vi "UNITEST MAIN v2.0.vi"() -> ()   [LabVIEW 2025] (continued)
      n79 = Bundle By Name(cluster=w163, "Loading.Enter the Loading Rate (N/min)"=w161, "Loading.Message"=w160, "Loading.Warning 2"=w159, "Loading.SSP 0.75"=w158, "Loading.SSP 0.5"=w157, "Loading.SSP 0.3"=w156, "Loading.Warning"=w155, "Loading.gui GIF"=w154, "Loading.Communication is established"=w153, "Loading.AppLoad 4"=w152, "Loading.Multipoint"=w151, "Loading.Indentation"=w150, "Loading.Reference Sample"=w149, "Loading.Load Cell Communication Slide"=w148, "Loading.com 3"=w147, "Loading.com"=w146, "Loading.DecaForce COM Status"=w145, "Loading.Update"=w144, "Loading.Clear 3"=w143, "Loading.seq"=w142, "Loading.Stribeck table"=w141, "Loading.Stribeck Table  For loading"=w140, "Loading.Loading Mode"=w139, "Loading.Enter the Final Load (N)"=w138, "Loading.Enter the CoF Trip"=w137, "Loading.Enter the Friction Force Trip"=w136, "Loading.Enter the Normal load Trip"=w135, "Loading.Enter the Load  (N)"=w134, "Loading.KiloForce"=w133, "Loading.DecaForce"=w132, "Loading.MicroForce"=w131, "Loading.LHBack"=w130, "Loading.LHNext"=w129, "Loading.Load Selection"=w128) -> (w162:T22)
    }
    frame #5 {
      n80 = control-ref of="TEST SELECTION"() -> (w215:refnum<vi>)
      n81 = control-ref of="SPEED SELECTION :"() -> (w214:refnum<vi>)
      n82 = control-ref of="SPEED SELECTION : rotary"() -> (w181:refnum<vi>)
      n83 = control-ref of="Rotary Tab"() -> (w230:refnum<vi>)
      n84 = control-ref of="e.v/ssr 2"() -> (w227:refnum<vi>)
      n85 = control-ref of="Step Speed"() -> (w211:refnum<vi>)
      n86 = control-ref of="M3 Image"() -> (w206:refnum<vi>)
      n87 = control-ref of="Rotary Module Selection"() -> (w183:refnum<vi>)
      n88 = control-ref of="zNL"() -> (w232:refnum<vi>)
      n89 = control-ref of="E.Velocity 2"() -> (w228:refnum<vi>)
      n90 = control-ref of="Ramp Up 2"() -> (w216:refnum<vi>)
      n91 = control-ref of="Angular Oscillation Set"() -> (w213:refnum<vi>)
      n92 = control-ref of="Traction"() -> (w212:refnum<vi>)
      n93 = control-ref of="Surge Forward MM"() -> (w208:refnum<vi>)
      n94 = control-ref of="Surge Backward MM"() -> (w207:refnum<vi>)
      n95 = control-ref of="Sway Left MM"() -> (w204:refnum<vi>)
      n96 = control-ref of="Sway Right MM"() -> (w203:refnum<vi>)
      n97 = control-ref of="Disable Axis Jog Soft Limits"() -> (w202:refnum<vi>)
      n98 = control-ref of="Heave Down MM"() -> (w200:refnum<vi>)
      n99 = control-ref of="Heave Up MM"() -> (w199:refnum<vi>)
      n100 = control-ref of="Set WTD"() -> (w197:refnum<vi>)
      n101 = control-ref of="HomeScratch"() -> (w196:refnum<vi>)
      n102 = control-ref of="HomeRot"() -> (w195:refnum<vi>)
      n103 = control-ref of="PlaceModule"() -> (w194:refnum<vi>)
      n104 = control-ref of="LR Sway"() -> (w190:refnum<vi>)
      n105 = control-ref of="Rot Hor"() -> (w189:refnum<vi>)
      n106 = control-ref of="Scratch"() -> (w188:refnum<vi>)
      n107 = control-ref of="LR Cam"() -> (w187:refnum<vi>)
      n108 = control-ref of="MMBack"() -> (w186:refnum<vi>)
      n109 = control-ref of="MMNext"() -> (w185:refnum<vi>)
      n110 = control-ref of="Rot Ver"() -> (w184:refnum<vi>)
      n111 = control-ref of="calculate rotary"() -> (w182:refnum<vi>)
      n112 = control-ref of="Import 2"() -> (w180:refnum<vi>)
      n113 = control-ref of="Save 2"() -> (w179:refnum<vi>)
      n114 = control-ref of="SwaySpeed Set"() -> (w172:refnum<vi>)
      n115 = control-ref of="HomeScratch"() -> (w168:refnum<vi>)
      n116 = control-ref of="NL disp"() -> (w231:refnum<vi>)
      n117 = control-ref of="Enter Fixed E.Velocity 2"() -> (w226:refnum<vi>)
      n118 = control-ref of="Enter Final SRR 2"() -> (w225:refnum<vi>)
      n119 = control-ref of="Enter initial SRR 2"() -> (w224:refnum<vi>)
      n120 = control-ref of="Enter Fixed SRR 2"() -> (w223:refnum<vi>)
      n121 = control-ref of="Enter the Final E.Velocity (m/s) 2"() -> (w222:refnum<vi>)
      n122 = control-ref of="Enter initial E.Velocity (m/s) 2"() -> (w221:refnum<vi>)
      n123 = control-ref of="Final Speed (RPM) 3"() -> (w220:refnum<vi>)
      n124 = control-ref of="Initial Speed (RPM) 2"() -> (w219:refnum<vi>)
      n125 = control-ref of="Enter the Final Velocity (m/s) 3"() -> (w218:refnum<vi>)
      n126 = control-ref of="Enter initial Velocity (m/s)  3"() -> (w217:refnum<vi>)
      n127 = control-ref of="mm"() -> (w201:refnum<vi>)
      n128 = control-ref of="Wear Track Diameter (mm)"() -> (w198:refnum<vi>)
      n129 = control-ref of="Enter the Angle (Deg)"() -> (w193:refnum<vi>)
      n130 = control-ref of="Enter the Frequency (Hz)"() -> (w192:refnum<vi>)
      n131 = control-ref of="Enter the Speed(mm/sec)"() -> (w175:refnum<vi>)
      n132 = control-ref of="Enter the Speed (RPM)"() -> (w174:refnum<vi>)
      n133 = control-ref of="Enter Scratch Speed (mm/s):"() -> (w173:refnum<vi>)
      n134 = control-ref of="Scartch Offset"() -> (w171:refnum<vi>)
      n135 = control-ref of="Enter Scratch length (mm):"() -> (w167:refnum<vi>)
      n136 = control-ref of="Wear Track Diameter"() -> (w166:refnum<vi>)
      n137 = control-ref of="No of Scratch"() -> (w164:refnum<vi>)
      n138 = control-ref of="String 39"() -> (w205:refnum<vi>)
      n139 = control-ref of="String 45"() -> (w177:refnum<vi>)
      n140 = control-ref of="Rotary Speed Exced"() -> (w165:refnum<vi>)
      n141 = control-ref of="StepTable For Load-Speed"() -> (w210:refnum<vi>)
      n142 = control-ref of="StepTable For Speed"() -> (w209:refnum<vi>)
      n143 = control-ref of="StepTable For Speed 3"() -> (w176:refnum<vi>)
      n144 = control-ref of="Motion Direction:  3"() -> (w229:refnum<vi>)
      n145 = control-ref of="Motion Mode:"() -> (w191:refnum<vi>)
      n146 = control-ref of="Scratch Mode"() -> (w170:refnum<vi>)
      n147 = control-ref of="Motion type:"() -> (w169:refnum<vi>)
      n148 = control-ref of="File Path :  2"() -> (w178:refnum<vi>)
      n149 = Bundle By Name(cluster=w234, "Motion Module.zNL"=w232, "Motion Module.NL disp"=w231, "Motion Module.Rotary Tab"=w230, "Motion Module.Motion Direction:  3"=w229, "Motion Module.E.Velocity 2"=w228, "Motion Module.e.v/ssr 2"=w227, "Motion Module.Enter Fixed E.Velocity 2"=w226, "Motion Module.Enter Final SRR 2"=w225, "Motion Module.Enter initial SRR 2"=w224, "Motion Module.Enter Fixed SRR 2"=w223, "Motion Module.Enter the Final E.Velocity (m/s) 2"=w222, "Motion Module.Enter initial E.Velocity (m/s) 2"=w221, "Motion Module.Final Speed (RPM) 3"=w220, "Motion Module.Initial Speed (RPM) 2"=w219, "Motion Module.Enter the Final Velocity (m/s) 3"=w218, "Motion Module.Enter initial Velocity (m/s)  3"=w217, "Motion Module.Ramp Up 2"=w216, "Motion Module.TEST SELECTION"=w215, "Motion Module.SPEED SELECTION :"=w214, "Motion Module.Angular Oscillation Set"=w213, "Motion Module.Traction"=w212, "Motion Module.Step Speed"=w211, "Motion Module.StepTable For Load-Speed"=w210, "Motion Module.StepTable For Speed"=w209, "Motion Module.Surge Forward MM"=w208, "Motion Module.Surge Backward MM"=w207, "Motion Module.M3 Image"=w206, "Motion Module.String 39"=w205, "Motion Module.Sway Left MM"=w204, "Motion Module.Sway Right MM"=w203, "Motion Module.Disable Axis Jog Soft Limits"=w202, "Motion Module.mm"=w201, "Motion Module.Heave Down MM"=w200, "Motion Module.Heave Up MM"=w199, "Motion Module.Wear Track Diameter (mm)"=w198, "Motion Module.Set WTD"=w197, "Motion Module.HomeScratch"=w196, "Motion Module.HomeRot"=w195, "Motion Module.PlaceModule"=w194, "Motion Module.Enter the Angle (Deg)"=w193, "Motion Module.Enter the Frequency (Hz)"=w192, "Motion Module.Motion Mode:"=w191, "Motion Module.LR Sway"=w190, "Motion Module.Rot Hor"=w189, "Motion Module.Scratch"=w188, "Motion Module.LR Cam"=w187, "Motion Module.MMBack"=w186, "Motion Module.MMNext"=w185, "Motion Module.Rot Ver"=w184, "Motion Module.Rotary Module Selection"=w183, "Motion Module.calculate rotary"=w182, "Motion Module.SPEED SELECTION : rotary"=w181, "Motion Module.Import 2"=w180, "Motion Module.Save 2"=w179, "Motion Module.File Path :  2"=w178, "Motion Module.String 45"=w177, "Motion Module.StepTable For Speed 3"=w176, "Motion Module.Enter the Speed(mm/sec)"=w175, "Motion Module.Enter the Speed(RPM)"=w174, "Motion Module.Enter Scratch Speed (mm/s):"=w173, "Motion Module.SwaySpeed Set"=w172, "Motion Module.Scartch Offset"=w171, "Motion Module.Scratch Mode"=w170, "Motion Module.Motion type:"=w169, "Motion Module.HomeScratch 2"=w168, "Motion Module.Enter Scratch length (mm):"=w167, "Motion Module.Wear Track Diameter"=w166, "Motion Module.Rotary Speed Exced"=w165, "Motion Module.No of Scratch"=w164) -> (w233:T22)
    }
    frame #6 {
      n150 = control-ref of="Add to list"() -> (w252:refnum<vi>)
      n151 = control-ref of="Wear"() -> (w251:refnum<vi>)
      n152 = control-ref of="Vibration"() -> (w250:refnum<vi>)
      n153 = control-ref of="Humidity (Chamber)"() -> (w249:refnum<vi>)
      n154 = control-ref of="Temperature (Chamber)"() -> (w248:refnum<vi>)
      n155 = control-ref of="ECR"() -> (w247:refnum<vi>)
      n156 = control-ref of="Temperature (Amb)"() -> (w246:refnum<vi>)
      n157 = control-ref of="Microphone"() -> (w245:refnum<vi>)
      n158 = control-ref of="Acoustic Emission 3"() -> (w244:refnum<vi>)
      n159 = control-ref of="SNext"() -> (w243:refnum<vi>)
      n160 = control-ref of="APBack"() -> (w242:refnum<vi>)
      n161 = control-ref of="Low Temp"() -> (w238:refnum<vi>)
      n162 = control-ref of="High Temp"() -> (w237:refnum<vi>)
      n163 = control-ref of="Humidity"() -> (w236:refnum<vi>)
      n164 = control-ref of="Humidity  Status  3"() -> (w259:refnum<vi>)
      n165 = control-ref of="Low Temp  Status  2"() -> (w258:refnum<vi>)
      n166 = control-ref of="TK4 status 2"() -> (w257:refnum<vi>)
      n167 = control-ref of="Humidity (Amb)"() -> (w254:refnum<vi>)
      n168 = control-ref of="Clear List"() -> (w253:refnum<vi>)
      n169 = control-ref of="Enter the Temperature (°C):"() -> (w241:refnum<vi>)
      n170 = control-ref of="Enter the Stage \nTemperature (°C):"() -> (w240:refnum<vi>)
      n171 = control-ref of="Enter the Humidity (%Rh):"() -> (w239:refnum<vi>)
      n172 = control-ref of="Sensors Picked"() -> (w235:refnum<vi>)
      n173 = control-ref of="Stage Temperature"() -> (w256:refnum<vi>)
      n174 = control-ref of="Sample Temperature"() -> (w255:refnum<vi>)
      n175 = Bundle By Name(cluster=w261, "Environmental control.Humidity  Status  3"=w259, "Environmental control.Low Temp  Status  2"=w258, "Environmental control.TK4 status 2"=w257, "Environmental control.Stage Temperature"=w256, "Environmental control.Sample Temperature"=w255, "Environmental control.Humidity (Amb)"=w254, "Environmental control.Clear List"=w253, "Environmental control.Add to list"=w252, "Environmental control.Wear"=w251, "Environmental control.Vibration"=w250, "Environmental control.Humidity (Chamber)"=w249, "Environmental control.Temperature (Chamber)"=w248, "Environmental control.ECR"=w247, "Environmental control.Temperature (Amb)"=w246, "Environmental control.Microphone"=w245, "Environmental control.Acoustic Emission 3"=w244, "Environmental control.SNext"=w243, "Environmental control.APBack"=w242, "Environmental control.Enter the Temperature (°C):"=w241, "Environmental control.Enter the Stage \nTemperature (°C):"=w240, "Environmental control.Enter the Humidity (%Rh):"=w239, "Environmental control.Low Temp"=w238, "Environmental control.High Temp"=w237, "Environmental control.Humidity"=w236, "Environmental control.Sensors Picked"=w235) -> (w260:T22)
    }
    frame #7 {
      n176 = control-ref of="ECR Port:"() -> (w271:refnum<vi>)
      n177 = control-ref of="Ramp Port:"() -> (w270:refnum<vi>)
      n178 = control-ref of="Heave and Surge COM Port:"() -> (w267:refnum<vi>)
      n179 = control-ref of="Sway COM Port:"() -> (w266:refnum<vi>)
      n180 = control-ref of="Temp Modbus:"() -> (w265:refnum<vi>)
      n181 = control-ref of="Humidity Port:"() -> (w264:refnum<vi>)
      n182 = control-ref of="About Tab"() -> (w272:refnum<vi>)
      n183 = control-ref of="Home Service"() -> (w274:refnum<vi>)
      n184 = control-ref of="Advanced Setting"() -> (w273:refnum<vi>)
      n185 = control-ref of="Installation/Replacement completed"() -> (w269:refnum<vi>)
      n186 = control-ref of="Loahead"() -> (w268:refnum<vi>)
      n187 = control-ref of="Edit Gain Constants"() -> (w263:refnum<vi>)
      n188 = control-ref of="Save Gain Constants"() -> (w262:refnum<vi>)
      n189 = control-ref of="Password"() -> (w275:refnum<vi>)
      n190 = Bundle By Name(cluster=w277, "About Screen.Password"=w275, "About Screen.Home Service"=w274, "About Screen.Advanced Setting"=w273, "About Screen.About Tab"=w272, "About Screen.ECR Port:"=w271, "About Screen.Ramp Port:"=w270, "About Screen.Installation/Replacement completed"=w269, "About Screen.Loahead"=w268, "About Screen.Heave and Surge COM Port:"=w267, "About Screen.Sway COM Port:"=w266, "About Screen.Temp Modbus:"=w265, "About Screen.Humidity Port:"=w264, "About Screen.Edit Gain Constants"=w263, "About Screen.Save Gain Constants"=w262) -> (w276:T22)
    }
    frame #8 {
      n191 = control-ref of="Cyclic Friction Force (N) Graph"() -> (w288:refnum<vi>)
      n192 = control-ref of="Cyclic Coefficient of Friction"() -> (w287:refnum<vi>)
      n193 = control-ref of="SDGp"() -> (w336:refnum<vi>)
      n194 = control-ref of="HumrGp"() -> (w334:refnum<vi>)
      n195 = control-ref of="gACQUOS"() -> (w331:refnum<vi>)
      n196 = control-ref of="ECR 2"() -> (w329:refnum<vi>)
      n197 = control-ref of="Temperature (deg c)"() -> (w327:refnum<vi>)
      n198 = control-ref of="MTM DISC  SPEED"() -> (w324:refnum<vi>)
      n199 = control-ref of="MTM BALL SPEED"() -> (w323:refnum<vi>)
      n200 = control-ref of="speed mm/sec"() -> (w322:refnum<vi>)
      n201 = control-ref of="WearGp"() -> (w312:refnum<vi>)
      n202 = control-ref of="Main Chart 3"() -> (w306:refnum<vi>)
      n203 = control-ref of="Friction Force (N) Graph"() -> (w294:refnum<vi>)
      n204 = control-ref of="Coefficient of Friction"() -> (w293:refnum<vi>)
      n205 = control-ref of="Main Screen Tab"() -> (w394:refnum<vi>)
      n206 = control-ref of="Angle and Frequency"() -> (w393:refnum<vi>)
      n207 = control-ref of="Main Speed Tab"() -> (w390:refnum<vi>)
      n208 = control-ref of="MTM MOTOR DISPLAY"() -> (w389:refnum<vi>)
      n209 = control-ref of="SPEED TAB"() -> (w384:refnum<vi>)
      n210 = control-ref of="Time Tab"() -> (w379:refnum<vi>)
      n211 = control-ref of="Temp Tabs"() -> (w372:refnum<vi>)
      n212 = control-ref of="Sub Graph"() -> (w339:refnum<vi>)
      n213 = control-ref of="Speed Tab"() -> (w325:refnum<vi>)
      n214 = control-ref of="FF Tab"() -> (w291:refnum<vi>)
      n215 = control-ref of="CZ FF"() -> (w289:refnum<vi>)
      n216 = control-ref of="Cyclic FF Disable Trip"() -> (w285:refnum<vi>)
      n217 = control-ref of="cyclic COF Disable Trip"() -> (w284:refnum<vi>)
      n218 = control-ref of="cyclic COF Reset Graph"() -> (w282:refnum<vi>)
      n219 = control-ref of="Cyclic FF Reset Graph"() -> (w281:refnum<vi>)
      n220 = control-ref of="Test Trip"() -> (w280:refnum<vi>)
      n221 = control-ref of="Scratch Start Test"() -> (w292:refnum<vi>)
      n222 = control-ref of="Scratch Start Recording"() -> (w278:refnum<vi>)
      n223 = control-ref of="Heater"() -> (w371:refnum<vi>)
      n224 = control-ref of="TK4 status"() -> (w370:refnum<vi>)
      n225 = control-ref of="Controller  Status"() -> (w367:refnum<vi>)
      n226 = control-ref of="Cooling"() -> (w364:refnum<vi>)
      n227 = control-ref of="Load Communication"() -> (w363:refnum<vi>)
      n228 = control-ref of="HumCOMStatus"() -> (w361:refnum<vi>)
      n229 = control-ref of="Load En"() -> (w358:refnum<vi>)
      n230 = control-ref of="NLt"() -> (w357:refnum<vi>)
      n231 = control-ref of="zNL 2"() -> (w356:refnum<vi>)
      n232 = control-ref of="Humidity On"() -> (w355:refnum<vi>)
      n233 = control-ref of="AppLoadSeq scratch"() -> (w351:refnum<vi>)
      n234 = control-ref of="Stop Scratch"() -> (w350:refnum<vi>)
      n235 = control-ref of="ClrLog"() -> (w349:refnum<vi>)
      n236 = control-ref of="STOP"() -> (w347:refnum<vi>)
      n237 = control-ref of="Start Test"() -> (w346:refnum<vi>)
      n238 = control-ref of="Test status"() -> (w345:refnum<vi>)
      n239 = control-ref of="AR Led"() -> (w344:refnum<vi>)
      n240 = control-ref of="Data"() -> (w343:refnum<vi>)
      n241 = control-ref of="Health"() -> (w342:refnum<vi>)
      n242 = control-ref of="Sway COM Status"() -> (w341:refnum<vi>)
      n243 = control-ref of="Heave COM Status"() -> (w340:refnum<vi>)
      n244 = control-ref of="Siliding distance Reset Graph"() -> (w337:refnum<vi>)
      n245 = control-ref of="Humidity Reset Graph"() -> (w335:refnum<vi>)
      n246 = control-ref of="Aqucostic Reset Graph"() -> (w332:refnum<vi>)
      n247 = control-ref of="ECR RESET"() -> (w330:refnum<vi>)
      n248 = control-ref of="Temperature Reset"() -> (w328:refnum<vi>)
      n249 = control-ref of="Speed Reset Graph"() -> (w326:refnum<vi>)
      n250 = control-ref of="Hymidity"() -> (w321:refnum<vi>)
      n251 = control-ref of="Humidity Disable trip"() -> (w320:refnum<vi>)
      n252 = control-ref of="Weart Deapth"() -> (w317:refnum<vi>)
      n253 = control-ref of="Depth Reset Graph"() -> (w316:refnum<vi>)
      n254 = control-ref of="Weart"() -> (w315:refnum<vi>)
      n255 = control-ref of="Depthz"() -> (w314:refnum<vi>)
      n256 = control-ref of="Load pid"() -> (w310:refnum<vi>)
      n257 = control-ref of="Load Disable Trip"() -> (w309:refnum<vi>)
      n258 = control-ref of="Load Reset Graph"() -> (w308:refnum<vi>)
      n259 = control-ref of="BACK"() -> (w305:refnum<vi>)
      n260 = control-ref of="zFF"() -> (w295:refnum<vi>)
      n261 = control-ref of="FF Reset Graph"() -> (w301:refnum<vi>)
      n262 = control-ref of="FF Disable Trip"() -> (w300:refnum<vi>)
      n263 = control-ref of="COF Disable Trip"() -> (w298:refnum<vi>)
      n264 = control-ref of="COF Reset Graph"() -> (w297:refnum<vi>)
      n265 = control-ref of="Start Test Temp"() -> (w296:refnum<vi>)
      n266 = control-ref of="Depth Trip 2"() -> (w304:refnum<vi>)
      n267 = control-ref of="Multi Scratch Pass"() -> (w279:refnum<vi>)
      n268 = control-ref of="Cyclic Friction Force (N)"() -> (w290:refnum<vi>)
      n269 = control-ref of="Cyclic FF TRIP"() -> (w286:refnum<vi>)
      n270 = control-ref of="cyclic COF TRIP"() -> (w283:refnum<vi>)
      n271 = control-ref of="Stroke (mm)"() -> (w392:refnum<vi>)
      n272 = control-ref of="Angle (Deg)"() -> (w391:refnum<vi>)
      n273 = control-ref of="Disc Speed (m/sec)"() -> (w388:refnum<vi>)
      n274 = control-ref of="Ball Speed (m/sec)"() -> (w387:refnum<vi>)
      n275 = control-ref of="Disc Speed (RPM)"() -> (w386:refnum<vi>)
      n276 = control-ref of="Ball Speed (RPM)"() -> (w385:refnum<vi>)
      n277 = control-ref of="Speed (m/sec)"() -> (w383:refnum<vi>)
      n278 = control-ref of="Set Speed (m/sec)"() -> (w382:refnum<vi>)
      n279 = control-ref of="Speed (RPM)"() -> (w381:refnum<vi>)
      n280 = control-ref of="Set Speed"() -> (w380:refnum<vi>)
      n281 = control-ref of="Time ( HH:MM:SS ) 2"() -> (w378:refnum<vi>)
      n282 = control-ref of="Test Duration"() -> (w377:refnum<vi>)
      n283 = control-ref of="Test Duration 4"() -> (w376:refnum<vi>)
      n284 = control-ref of="TEST CYCLE"() -> (w375:refnum<vi>)
      n285 = control-ref of="TOTAL CYCLES"() -> (w374:refnum<vi>)
      n286 = control-ref of="Set Load (N)"() -> (w373:refnum<vi>)
      n287 = control-ref of="ChamberTemp"() -> (w369:refnum<vi>)
      n288 = control-ref of="SetTmp"() -> (w368:refnum<vi>)
      n289 = control-ref of="ChamberTemp"() -> (w366:refnum<vi>)
      n290 = control-ref of="SetTmp"() -> (w365:refnum<vi>)
      n291 = control-ref of="Ambient \nTemperature"() -> (w362:refnum<vi>)
      n292 = control-ref of="Ambient\n Humidity"() -> (w360:refnum<vi>)
      n293 = control-ref of="Freq (Hz)"() -> (w359:refnum<vi>)
      n294 = control-ref of="humidity disp"() -> (w354:refnum<vi>)
      n295 = control-ref of="Set Humidity"() -> (w353:refnum<vi>)
      n296 = control-ref of="NL disp 2"() -> (w352:refnum<vi>)
      n297 = control-ref of="SD (mm)"() -> (w338:refnum<vi>)
      n298 = control-ref of="Acoustic Emission (mV)"() -> (w333:refnum<vi>)
      n299 = control-ref of="CoF Trip  2"() -> (w319:refnum<vi>)
      n300 = control-ref of="Depth Trip"() -> (w318:refnum<vi>)
      n301 = control-ref of="Depth (µm)"() -> (w313:refnum<vi>)
      n302 = control-ref of="NL Trip 2"() -> (w311:refnum<vi>)
      n303 = control-ref of="NL Display 4"() -> (w307:refnum<vi>)
      n304 = control-ref of="COF TRIP"() -> (w303:refnum<vi>)
      n305 = control-ref of="Friction Force (N)"() -> (w302:refnum<vi>)
      n306 = control-ref of="FF TRIP"() -> (w299:refnum<vi>)
      n307 = control-ref of="Trip Log"() -> (w348:refnum<vi>)
      n308 = Bundle By Name(cluster=w396, "Main Screen.Test Trip"=w280, "Main Screen.Main Screen Tab"=w394, "Main Screen.Angle and Frequency"=w393, "Main Screen.Stroke (mm)"=w392, "Main Screen.Angle (Deg)"=w391, "Main Screen.Main Speed Tab"=w390, "Main Screen.MTM MOTOR DISPLAY"=w389, "Main Screen.Disc Speed (m/sec)"=w388, "Main Screen.Ball Speed (m/sec)"=w387, "Main Screen.Disc Speed (RPM)"=w386, "Main Screen.Ball Speed (RPM)"=w385, "Main Screen.SPEED TAB"=w384, "Main Screen.Speed (m/sec)"=w383, "Main Screen.Set Speed (m/sec)"=w382, "Main Screen.Speed (RPM)"=w381, "Main Screen.Set Speed"=w380, "Main Screen.Time Tab"=w379, "Main Screen.Time ( HH:MM:SS ) 2"=w378, "Main Screen.Test Duration"=w377, "Main Screen.Test Duration 4"=w376, "Main Screen.TEST CYCLE"=w375, "Main Screen.TOTAL CYCLES"=w374, "Main Screen.Set Load (N)"=w373, "Main Screen.Temp Tabs"=w372, "Main Screen.Heater"=w371, "Main Screen.TK4 status"=w370, "Main Screen.ChamberTemp"=w369, "Main Screen.SetTmp"=w368, "Main Screen.Controller  Status"=w367, "Main Screen.ChamberTemp 2"=w366, "Main Screen.SetTmp 2"=w365, "Main Screen.Cooling"=w364, "Main Screen.Load Communication"=w363, "Main Screen.Ambient \nTemperature"=w362, "Main Screen.HumCOMStatus"=w361, "Main Screen.Ambient\n Humidity"=w360, "Main Screen.Freq (Hz)"=w359, "Main Screen.Load En"=w358, "Main Screen.NLt"=w357, "Main Screen.zNL 2"=w356, "Main Screen.Humidity On"=w355, "Main Screen.humidity disp"=w354, "Main Screen.Set Humidity"=w353, "Main Screen.NL disp 2"=w352, "Main Screen.AppLoadSeq scratch"=w351, "Main Screen.Stop Scratch"=w350, "Main Screen.ClrLog"=w349, "Main Screen.Trip Log"=w348, "Main Screen.STOP"=w347, "Main Screen.Start Test"=w346, "Main Screen.Test status"=w345, "Main Screen.AR Led"=w344, "Main Screen.Data"=w343, "Main Screen.Health"=w342, "Main Screen.Sway COM Status"=w341, "Main Screen.Heave COM Status"=w340, "Main Screen.Sub Graph"=w339, "Main Screen.SD (mm)"=w338, "Main Screen.Siliding distance Reset Graph"=w337, "Main Screen.SDGp"=w336, "Main Screen.Humidity Reset Graph"=w335, "Main Screen.HumrGp"=w334, "Main Screen.Acoustic Emission (mV)"=w333, "Main Screen.Aqucostic Reset Graph"=w332, "Main Screen.gACQUOS"=w331, "Main Screen.ECR RESET"=w330, "Main Screen.ECR"=w329, "Main Screen.Temperature Reset"=w328, "Main Screen.Temperature (deg c)"=w327, "Main Screen.Speed Reset Graph"=w326, "Main Screen.Speed Tab"=w325, "Main Screen.MTM DISC  SPEED"=w324, "Main Screen.MTM BALL SPEED"=w323, "Main Screen.speed mm/sec"=w322, "Main Screen.Hymidity"=w321, "Main Screen.Humidity Disable trip"=w320, "Main Screen.CoF Trip  2"=w319, "Main Screen.Depth Trip"=w318, "Main Screen.Weart Deapth"=w317, "Main Screen.Depth Reset Graph"=w316, "Main Screen.Weart"=w315, "Main Screen.Depthz"=w314, "Main Screen.Depth (µm)"=w313, "Main Screen.WearGp"=w312, "Main Screen.NL Trip 2"=w311, "Main Screen.Load pid"=w310, "Main Screen.Load Disable Trip"=w309, "Main Screen.Load Reset Graph"=w308, "Main Screen.NL Display 4"=w307, "Main Screen.Main Chart 3"=w306, "Main Screen.BACK"=w305, "Main Screen.Depth Trip 2"=w304, "Main Screen.COF TRIP"=w303, "Main Screen.Friction Force (N)"=w302, "Main Screen.FF Reset Graph"=w301, "Main Screen.FF Disable Trip"=w300, "Main Screen.FF TRIP"=w299, "Main Screen.COF Disable Trip"=w298, "Main Screen.COF Reset Graph"=w297, "Main Screen.FF Tab"=w291, "Main Screen.Start Test Temp"=w296, "Main Screen.zFF"=w295, "Main Screen.Friction Force (N) Graph"=w294, "Main Screen.Coefficient of Friction"=w293, "Main Screen.Scratch Start Test"=w292, "Main Screen.Cyclic Friction Force (N)"=w290, "Main Screen.CZ FF"=w289, "Main Screen.Cyclic Friction Force (N) Graph"=w288, "Main Screen.Cyclic Coefficient of Friction"=w287, "Main Screen.Cyclic FF TRIP"=w286, "Main Screen.Cyclic FF Disable Trip"=w285, "Main Screen.cyclic COF Disable Trip"=w284, "Main Screen.cyclic COF TRIP"=w283, "Main Screen.cyclic COF Reset Graph"=w282, "Main Screen.Cyclic FF Reset Graph"=w281, "Main Screen.Multi Scratch Pass"=w279, "Main Screen.Scratch Start Recording"=w278) -> (w395:T22)
    }
    frame #9 {
      n309 = control-ref of="gFF Rot 7"() -> (w400:refnum<vi>)
      n310 = control-ref of="Ramp"() -> (w419:refnum<vi>)
      n311 = control-ref of="Dummy Run"() -> (w413:refnum<vi>)
      n312 = control-ref of="AutoTune"() -> (w411:refnum<vi>)
      n313 = control-ref of="apply load"() -> (w409:refnum<vi>)
      n314 = control-ref of="reinit 3"() -> (w407:refnum<vi>)
      n315 = control-ref of="Bypass Load"() -> (w404:refnum<vi>)
      n316 = control-ref of="PID gains out delay (microForce)"() -> (w420:refnum<vi>)
      n317 = control-ref of="output range delay"() -> (w406:refnum<vi>)
      n318 = control-ref of="PID gains out delay"() -> (w405:refnum<vi>)
      n319 = control-ref of="Ramp MulFac"() -> (w424:refnum<vi>)
      n320 = control-ref of="pulses LoadDiffRamp(2..10)"() -> (w423:refnum<vi>)
      n321 = control-ref of="PulseControlRamp(diff<=3N)"() -> (w422:refnum<vi>)
      n322 = control-ref of="SetLoadDeadband(%) Load(0-10N)"() -> (w421:refnum<vi>)
      n323 = control-ref of="Gain 2"() -> (w418:refnum<vi>)
      n324 = control-ref of="pulses LoadDiff(2..10)"() -> (w417:refnum<vi>)
      n325 = control-ref of="pulses LoadDiff(11..50)"() -> (w416:refnum<vi>)
      n326 = control-ref of="PulseControl(diff<=3N)"() -> (w415:refnum<vi>)
      n327 = control-ref of="SetLoadDeadband(%)  2"() -> (w414:refnum<vi>)
      n328 = control-ref of="Vertical load (N)"() -> (w412:refnum<vi>)
      n329 = control-ref of="Offset  3"() -> (w410:refnum<vi>)
      n330 = control-ref of="Enter ByPass Load"() -> (w408:refnum<vi>)
      n331 = control-ref of="pulsesSent"() -> (w403:refnum<vi>)
      n332 = control-ref of="pulses"() -> (w402:refnum<vi>)
      n333 = control-ref of="actpid"() -> (w401:refnum<vi>)
      n334 = control-ref of="pulses LoadDiff(21..1000)"() -> (w399:refnum<vi>)
      n335 = control-ref of="Delay"() -> (w398:refnum<vi>)
      n336 = control-ref of="deadband"() -> (w397:refnum<vi>)
      n337 = Bundle By Name(cluster=w426, "PID.Ramp MulFac"=w424, "PID.pulses LoadDiffRamp(2..10)"=w423, "PID.PulseControlRamp(diff<=3N)"=w422, "PID.SetLoadDeadband(%) Load(0-10N)"=w421, "PID.PID gains out delay (microForce)"=w420, "PID.Ramp"=w419, "PID.Gain 2"=w418, "PID.pulses LoadDiff(2..10)"=w417, "PID.pulses LoadDiff(11..50)"=w416, "PID.PulseControl(diff<=3N)"=w415, "PID.SetLoadDeadband(%)  2"=w414, "PID.Dummy Run"=w413, "PID.Vertical load (N)"=w412, "PID.AutoTune"=w411, "PID.Offset 3"=w410, "PID.apply load"=w409, "PID.Enter ByPass Load"=w408, "PID.reinit 3"=w407, "PID.output range delay"=w406, "PID.PID gains out delay"=w405, "PID.Bypass Load"=w404, "PID.pulsesSent"=w403, "PID.pulses"=w402, "PID.actpid"=w401, "PID.gFF Rot"=w400, "PID.pulses LoadDiff(21..1000)"=w399, "PID.Delay"=w398, "PID.deadband"=w397) -> (w425:T22)
    }
    frame #10 {
      n338 = control-ref of="Tab Control 3"() -> (w494:refnum<vi>)
      n339 = control-ref of="Tab Control 19"() -> (w493:refnum<vi>)
      n340 = control-ref of="Tab Control 14"() -> (w454:refnum<vi>)
      n341 = control-ref of="DEPTH TRIP   ENABLE"() -> (w443:refnum<vi>)
      n342 = control-ref of="LOAD TRIP  ENABLE"() -> (w442:refnum<vi>)
      n343 = control-ref of="CYCLIC COF TRIP  ENABLE"() -> (w437:refnum<vi>)
      n344 = control-ref of="CYCLIC FF TRIP  ENABLE"() -> (w436:refnum<vi>)
      n345 = control-ref of="FF TRIP  ENABLE"() -> (w435:refnum<vi>)
      n346 = control-ref of="COF TRIP  ENABLE"() -> (w434:refnum<vi>)
      n347 = control-ref of="Rotary Vertical"() -> (w432:refnum<vi>)
      n348 = control-ref of="Traction"() -> (w431:refnum<vi>)
      n349 = control-ref of="Scratch"() -> (w430:refnum<vi>)
      n350 = control-ref of="LRM CAM"() -> (w429:refnum<vi>)
      n351 = control-ref of="Sway LRM"() -> (w428:refnum<vi>)
      n352 = control-ref of="Rotary Horizontal"() -> (w427:refnum<vi>)
      n353 = control-ref of="Re-initilaize"() -> (w491:refnum<vi>)
      n354 = control-ref of="Filter ON/OFF"() -> (w490:refnum<vi>)
      n355 = control-ref of="Apply Filter (FF)"() -> (w486:refnum<vi>)
      n356 = control-ref of="Apply Filter (Load)"() -> (w484:refnum<vi>)
      n357 = control-ref of="SAVE  2"() -> (w479:refnum<vi>)
      n358 = control-ref of="Enter Distance"() -> (w478:refnum<vi>)
      n359 = control-ref of="AE"() -> (w453:refnum<vi>)
      n360 = control-ref of="Heave Loop Delay"() -> (w452:refnum<vi>)
      n361 = control-ref of="Heave PID Speed"() -> (w451:refnum<vi>)
      n362 = control-ref of="Surge Jog Speed"() -> (w450:refnum<vi>)
      n363 = control-ref of="Heave Jog Speed"() -> (w449:refnum<vi>)
      n364 = control-ref of="Sway Loop Delay"() -> (w448:refnum<vi>)
      n365 = control-ref of="Sway PID Speed"() -> (w447:refnum<vi>)
      n366 = control-ref of="Sway Jog Speed"() -> (w446:refnum<vi>)
      n367 = control-ref of="DEPTH TRIP VALUE"() -> (w445:refnum<vi>)
      n368 = control-ref of="LOAD TRIP VALUE"() -> (w444:refnum<vi>)
      n369 = control-ref of="CYCLIC FF TRIP VALUE"() -> (w441:refnum<vi>)
      n370 = control-ref of="FF TRIP VALUE"() -> (w440:refnum<vi>)
      n371 = control-ref of="CYCLIC CoF TRIP VALUE"() -> (w439:refnum<vi>)
      n372 = control-ref of="COF TRIP VALUE"() -> (w438:refnum<vi>)
      n373 = control-ref of="JOG TRIP LOAD VALUE (N)"() -> (w433:refnum<vi>)
      n374 = control-ref of="SAMPLES"() -> (w492:refnum<vi>)
      n375 = control-ref of="TracHomeSurgeOffsetCounts 10MM"() -> (w489:refnum<vi>)
      n376 = control-ref of="TracHomeSwayOffsetCounts 10MM"() -> (w488:refnum<vi>)
      n377 = control-ref of="Acoustic Emission:"() -> (w487:refnum<vi>)
      n378 = control-ref of="Filter% 2"() -> (w485:refnum<vi>)
      n379 = control-ref of="Filter%"() -> (w483:refnum<vi>)
      n380 = control-ref of="Sway distance (mm)"() -> (w482:refnum<vi>)
      n381 = control-ref of="Surge distance (mm)"() -> (w481:refnum<vi>)
      n382 = control-ref of="DataSavingLoopDelay(ms)"() -> (w480:refnum<vi>)
      n383 = control-ref of="Sway Counts:"() -> (w477:refnum<vi>)
      n384 = control-ref of="Distance (mm): 3"() -> (w476:refnum<vi>)
      n385 = control-ref of="Surge Counts:"() -> (w475:refnum<vi>)
      n386 = control-ref of="Distance (mm): 2"() -> (w474:refnum<vi>)
      n387 = control-ref of="Distance (mm):"() -> (w473:refnum<vi>)
      n388 = control-ref of="Heave Counts:"() -> (w472:refnum<vi>)
      n389 = control-ref of="LRMHomeSurgeOffsetCounts"() -> (w471:refnum<vi>)
      n390 = control-ref of="LRMHomeSwayOffsetCounts"() -> (w470:refnum<vi>)
      n391 = control-ref of="TracHomeSurgeOffsetCounts 20MM"() -> (w469:refnum<vi>)
      n392 = control-ref of="TracHomeSwayOffsetCounts 20MM"() -> (w468:refnum<vi>)
      n393 = control-ref of="RotHomeSwayOffsetCounts"() -> (w467:refnum<vi>)
      n394 = control-ref of="RotHomeSurgeOffsetCounts"() -> (w466:refnum<vi>)
      n395 = control-ref of="Heave distance"() -> (w465:refnum<vi>)
      n396 = control-ref of="Zmm"() -> (w464:refnum<vi>)
      n397 = control-ref of="Heave Pulses/mm"() -> (w463:refnum<vi>)
      n398 = control-ref of="Surge Pulses/mm"() -> (w462:refnum<vi>)
      n399 = control-ref of="Sway Pulses/mm"() -> (w461:refnum<vi>)
      n400 = control-ref of="Heave Pitch"() -> (w460:refnum<vi>)
      n401 = control-ref of="Surge Pitch"() -> (w459:refnum<vi>)
      n402 = control-ref of="Sway Pitch"() -> (w458:refnum<vi>)
      n403 = control-ref of="Heave PPR"() -> (w457:refnum<vi>)
      n404 = control-ref of="Surge PPR"() -> (w456:refnum<vi>)
      n405 = control-ref of="Sway PPR"() -> (w455:refnum<vi>)
      n406 = Bundle By Name(cluster=w496, "Config Parameters.Tab Control 3"=w494, "Config Parameters.Tab Control 19"=w493, "Config Parameters.SAMPLES"=w492, "Config Parameters.Re-initilaize"=w491, "Config Parameters.Filter ON/OFF"=w490, "Config Parameters.TracHomeSurgeOffsetCounts 10MM"=w489, "Config Parameters.TracHomeSwayOffsetCounts 10MM"=w488, "Config Parameters.Acoustic Emission:"=w487, "Config Parameters.Apply Filter (FF)"=w486, "Config Parameters.Filter% 2"=w485, "Config Parameters.Apply Filter (Load)"=w484, "Config Parameters.Filter%"=w483, "Config Parameters.Sway distance (mm)"=w482, "Config Parameters.Surge distance (mm)"=w481, "Config Parameters.DataSavingLoopDelay(ms)"=w480, "Config Parameters.SAVE 2"=w479, "Config Parameters.Enter Distance"=w478, "Config Parameters.Sway Counts:"=w477, "Config Parameters.Distance (mm): 3"=w476, "Config Parameters.Surge Counts:"=w475, "Config Parameters.Distance (mm): 2"=w474, "Config Parameters.Distance (mm):"=w473, "Config Parameters.Heave Counts:"=w472, "Config Parameters.LRMHomeSurgeOffsetCounts"=w471, "Config Parameters.LRMHomeSwayOffsetCounts"=w470, "Config Parameters.TracHomeSurgeOffsetCounts 20MM"=w469, "Config Parameters.TracHomeSwayOffsetCounts 20MM"=w468, "Config Parameters.RotHomeSwayOffsetCounts"=w467, "Config Parameters.RotHomeSurgeOffsetCounts"=w466, "Config Parameters.Heave distance"=w465, "Config Parameters.Zmm"=w464, "Config Parameters.Heave Pulses/mm"=w463, "Config Parameters.Surge Pulses/mm"=w462, "Config Parameters.Sway Pulses/mm"=w461, "Config Parameters.Heave Pitch"=w460, "Config Parameters.Surge Pitch"=w459, "Config Parameters.Sway Pitch"=w458, "Config Parameters.Heave PPR"=w457, "Config Parameters.Surge PPR"=w456, "Config Parameters.Sway PPR"=w455, "Config Parameters.Tab Control 14"=w454, "Config Parameters.AE"=w453, "Config Parameters.Heave Loop Delay"=w452, "Config Parameters.Heave PID Speed"=w451, "Config Parameters.Surge Jog Speed"=w450, "Config Parameters.Heave Jog Speed"=w449, "Config Parameters.Sway Loop Delay"=w448, "Config Parameters.Sway PID Speed"=w447, "Config Parameters.Sway Jog Speed"=w446, "Config Parameters.DEPTH TRIP VALUE"=w445, "Config Parameters.LOAD TRIP VALUE"=w444, "Config Parameters.DEPTH TRIP   ENABLE"=w443, "Config Parameters.LOAD TRIP  ENABLE"=w442, "Config Parameters.CYCLIC FF TRIP VALUE"=w441, "Config Parameters.FF TRIP VALUE"=w440, "Config Parameters.CYCLIC CoF TRIP VALUE"=w439, "Config Parameters.COF TRIP VALUE"=w438, "Config Parameters.CYCLIC COF TRIP  ENABLE"=w437, "Config Parameters.CYCLIC FF TRIP  ENABLE"=w436, "Config Parameters.FF TRIP  ENABLE"=w435, "Config Parameters.COF TRIP  ENABLE"=w434, "Config Parameters.JOG TRIP LOAD VALUE (N)"=w433, "Config Parameters.Rotary Vertical"=w432, "Config Parameters.Traction"=w431, "Config Parameters.Scratch"=w430, "Config Parameters.LRM CAM"=w429, "Config Parameters.Sway LRM"=w428, "Config Parameters.Rotary Horizontal"=w427) -> (w495:T22)
    }
    frame #11 {
      n407 = control-ref of="FORCE (N)"() -> (w498:refnum<vi>)
      n408 = control-ref of="TORQUE (N-m)"() -> (w497:refnum<vi>)
      n409 = control-ref of="Load Cell Temp"() -> (w499:refnum<vi>)
      n410 = control-ref of="ClearAll"() -> (w527:refnum<vi>)
      n411 = control-ref of="ZeroAll"() -> (w522:refnum<vi>)
      n412 = control-ref of="delete Handle"() -> (w512:refnum<vi>)
      n413 = control-ref of="Create Handle"() -> (w511:refnum<vi>)
      n414 = control-ref of="stop 6"() -> (w508:refnum<vi>)
      n415 = control-ref of="running_flag"() -> (w507:refnum<vi>)
      n416 = control-ref of="Save Dwell"() -> (w523:refnum<vi>)
      n417 = control-ref of="Acq Delay (ms)"() -> (w521:refnum<vi>)
      n418 = control-ref of="Burst Delay (ms)"() -> (w520:refnum<vi>)
      n419 = control-ref of="SN"() -> (w518:refnum<vi>)
      n420 = control-ref of="Port"() -> (w515:refnum<vi>)
      n421 = control-ref of="ft_udp_handle"() -> (w506:refnum<vi>)
      n422 = control-ref of="get-data-return"() -> (w505:refnum<vi>)
      n423 = control-ref of="get-range-return"() -> (w504:refnum<vi>)
      n424 = control-ref of="zero-return"() -> (w503:refnum<vi>)
      n425 = control-ref of="filter-return"() -> (w502:refnum<vi>)
      n426 = control-ref of="initial-return"() -> (w501:refnum<vi>)
      n427 = control-ref of="deleteHandle-result"() -> (w500:refnum<vi>)
      n428 = control-ref of="model"() -> (w519:refnum<vi>)
      n429 = control-ref of="Sensor IP"() -> (w516:refnum<vi>)
      n430 = control-ref of="Mz(Nm)"() -> (w526:refnum<vi>)
      n431 = control-ref of="My(Nm)"() -> (w525:refnum<vi>)
      n432 = control-ref of="Mx(Nm)"() -> (w524:refnum<vi>)
      n433 = control-ref of="FFx(N)"() -> (w517:refnum<vi>)
      n434 = control-ref of="FFy(N)"() -> (w514:refnum<vi>)
      n435 = control-ref of="Load(N)"() -> (w513:refnum<vi>)
      n436 = control-ref of="ft_data"() -> (w510:refnum<vi>)
      n437 = control-ref of="ft_range"() -> (w509:refnum<vi>)
      n438 = Bundle By Name(cluster=w529, "Loading Com Port.ClearAll"=w527, "Loading Com Port.Mz(Nm)"=w526, "Loading Com Port.My(Nm)"=w525, "Loading Com Port.Mx(Nm)"=w524, "Loading Com Port.Save Dwell"=w523, "Loading Com Port.ZeroAll"=w522, "Loading Com Port.Acq Delay (ms)"=w521, "Loading Com Port.Burst Delay (ms)"=w520, "Loading Com Port.model"=w519, "Loading Com Port.SN"=w518, "Loading Com Port.FFx(N)"=w517, "Loading Com Port.Sensor IP"=w516, "Loading Com Port.Port"=w515, "Loading Com Port.FFy(N)"=w514, "Loading Com Port.Load(N)"=w513, "Loading Com Port.delete Handle"=w512, "Loading Com Port.Create Handle"=w511, "Loading Com Port.ft_data"=w510, "Loading Com Port.ft_range"=w509, "Loading Com Port.stop 6"=w508, "Loading Com Port.running_flag"=w507, "Loading Com Port.ft_udp_handle"=w506, "Loading Com Port.get-data-return"=w505, "Loading Com Port.get-range-return"=w504, "Loading Com Port.zero-return"=w503, "Loading Com Port.filter-return"=w502, "Loading Com Port.initial-return"=w501, "Loading Com Port.deleteHandle-result"=w500, "Loading Com Port.Load Cell Temp"=w499, "Loading Com Port.FORCE (N)"=w498, "Loading Com Port.TORQUE (N-m)"=w497) -> (w528:T22)
    }
    frame #12 {
      n439 = control-ref of="Read Heave Temp"() -> (w575:refnum<vi>)
      n440 = control-ref of="Manual Write Heave & Surge"() -> (w552:refnum<vi>)
      n441 = control-ref of="error out Read"() -> (w587:refnum<vi>)
      n442 = control-ref of="error out Write"() -> (w582:refnum<vi>)
      n443 = control-ref of="UPLINK HEAVE"() -> (w531:refnum<vi>)
      n444 = control-ref of="DOWNLINK HEAVE"() -> (w530:refnum<vi>)
      n445 = control-ref of="SURGE POSE"() -> (w588:refnum<vi>)
      n446 = control-ref of="HEAVE POSE"() -> (w586:refnum<vi>)
      n447 = control-ref of="State"() -> (w585:refnum<vi>)
      n448 = control-ref of="Homed"() -> (w584:refnum<vi>)
      n449 = control-ref of="Sequence ID"() -> (w583:refnum<vi>)
      n450 = control-ref of="faultCode"() -> (w581:refnum<vi>)
      n451 = control-ref of="Ack ID"() -> (w580:refnum<vi>)
      n452 = control-ref of="SPEED"() -> (w579:refnum<vi>)
      n453 = control-ref of="Distance"() -> (w578:refnum<vi>)
      n454 = control-ref of="Mode Command"() -> (w577:refnum<vi>)
      n455 = control-ref of="SPARE 2"() -> (w574:refnum<vi>)
      n456 = control-ref of="SPARE 1"() -> (w573:refnum<vi>)
      n457 = control-ref of="Spare 15"() -> (w572:refnum<vi>)
      n458 = control-ref of="Spare 14"() -> (w571:refnum<vi>)
      n459 = control-ref of="Spare 13"() -> (w570:refnum<vi>)
      n460 = control-ref of="Spare 12"() -> (w569:refnum<vi>)
      n461 = control-ref of="Spare 11"() -> (w568:refnum<vi>)
      n462 = control-ref of="Spare 10"() -> (w567:refnum<vi>)
      n463 = control-ref of="Spare 9"() -> (w566:refnum<vi>)
      n464 = control-ref of="Spare 8"() -> (w565:refnum<vi>)
      n465 = control-ref of="Spare 7"() -> (w564:refnum<vi>)
      n466 = control-ref of="Spare 6"() -> (w563:refnum<vi>)
      n467 = control-ref of="Spare 5"() -> (w562:refnum<vi>)
      n468 = control-ref of="Spare 4"() -> (w561:refnum<vi>)
      n469 = control-ref of="Spare 3"() -> (w560:refnum<vi>)
      n470 = control-ref of="Spare 2"() -> (w559:refnum<vi>)
      n471 = control-ref of="Spare 1"() -> (w558:refnum<vi>)
      n472 = control-ref of="Node Id"() -> (w557:refnum<vi>)
      n473 = control-ref of="SPARE 3"() -> (w556:refnum<vi>)
      n474 = control-ref of="SPARE 4"() -> (w555:refnum<vi>)
      n475 = control-ref of="fwMajor"() -> (w554:refnum<vi>)
      n476 = control-ref of="fwMinor"() -> (w553:refnum<vi>)
      n477 = control-ref of="SPARE 5"() -> (w550:refnum<vi>)
      n478 = control-ref of="Reserved"() -> (w549:refnum<vi>)
      n479 = control-ref of="SPARE 8"() -> (w548:refnum<vi>)
      n480 = control-ref of="SPARE 6"() -> (w547:refnum<vi>)
      n481 = control-ref of="SPARE 7"() -> (w546:refnum<vi>)
      n482 = control-ref of="SPARE 17"() -> (w545:refnum<vi>)
      n483 = control-ref of="SPARE 16"() -> (w544:refnum<vi>)
      n484 = control-ref of="SPARE 15"() -> (w543:refnum<vi>)
      n485 = control-ref of="SPARE 14"() -> (w542:refnum<vi>)
      n486 = control-ref of="SPARE 13"() -> (w541:refnum<vi>)
      n487 = control-ref of="SPARE 12"() -> (w540:refnum<vi>)
      n488 = control-ref of="SPARE 11"() -> (w539:refnum<vi>)
      n489 = control-ref of="SPARE 10"() -> (w538:refnum<vi>)
      n490 = control-ref of="SPARE 9"() -> (w537:refnum<vi>)
      n491 = control-ref of="System UPTIME"() -> (w536:refnum<vi>)
      n492 = control-ref of="Missed Packets"() -> (w535:refnum<vi>)
      n493 = control-ref of="faultCode Surge Right"() -> (w534:refnum<vi>)
      n494 = control-ref of="faultCode Surge Left"() -> (w533:refnum<vi>)
      n495 = control-ref of="faultCode Heave"() -> (w532:refnum<vi>)
      n496 = control-ref of="Heave and Surge Read"() -> (w576:refnum<vi>)
      n497 = control-ref of="Heave and Surge Write"() -> (w551:refnum<vi>)
      n498 = Bundle By Name(cluster=w590, "Heave AND Surge.SURGE POSE"=w588, "Heave AND Surge.error out Read"=w587, "Heave AND Surge.HEAVE POSE"=w586, "Heave AND Surge.State"=w585, "Heave AND Surge.Homed"=w584, "Heave AND Surge.Sequence ID"=w583, "Heave AND Surge.error out Write"=w582, "Heave AND Surge.faultCode"=w581, "Heave AND Surge.Ack ID"=w580, "Heave AND Surge.SPEED"=w579, "Heave AND Surge.Distance"=w578, "Heave AND Surge.Mode Command"=w577, "Heave AND Surge.Heave and Surge Read"=w576, "Heave AND Surge.Read Heave Temp"=w575, "Heave AND Surge.SPARE 2"=w574, "Heave AND Surge.SPARE 1"=w573, "Heave AND Surge.Spare 15"=w572, "Heave AND Surge.Spare 14"=w571, "Heave AND Surge.Spare 13"=w570, "Heave AND Surge.Spare 12"=w569, "Heave AND Surge.Spare 11"=w568, "Heave AND Surge.Spare 10"=w567, "Heave AND Surge.Spare 9"=w566, "Heave AND Surge.Spare 8"=w565, "Heave AND Surge.Spare 7"=w564, "Heave AND Surge.Spare 6"=w563, "Heave AND Surge.Spare 5"=w562, "Heave AND Surge.Spare 4"=w561, "Heave AND Surge.Spare 3"=w560, "Heave AND Surge.Spare 2"=w559, "Heave AND Surge.Spare 1"=w558, "Heave AND Surge.Node Id"=w557, "Heave AND Surge.SPARE 3"=w556, "Heave AND Surge.SPARE 4"=w555, "Heave AND Surge.fwMajor"=w554, "Heave AND Surge.fwMinor"=w553, "Heave AND Surge.Manual Write"=w552, "Heave AND Surge.Heave and Surge Write"=w551, "Heave AND Surge.SPARE 5"=w550, "Heave AND Surge.Reserved"=w549, "Heave AND Surge.SPARE 8"=w548, "Heave AND Surge.SPARE 6"=w547, "Heave AND Surge.SPARE 7"=w546, "Heave AND Surge.SPARE 17"=w545, "Heave AND Surge.SPARE 16"=w544, "Heave AND Surge.SPARE 15"=w543, "Heave AND Surge.SPARE 14"=w542, "Heave AND Surge.SPARE 13"=w541, "Heave AND Surge.SPARE 12"=w540, "Heave AND Surge.SPARE 11"=w539, "Heave AND Surge.SPARE 10"=w538, "Heave AND Surge.SPARE 9"=w537, "Heave AND Surge.System UPTIME"=w536, "Heave AND Surge.Missed Packets"=w535, "Heave AND Surge.faultCode Surge Right"=w534, "Heave AND Surge.faultCode Surge Left"=w533, "Heave AND Surge.faultCode Heave"=w532, "Heave AND Surge.UPLINK HEAVE"=w531, "Heave AND Surge.DOWNLINK HEAVE"=w530) -> (w589:T22)
    }
    frame #13 {
      n499 = control-ref of="PID"() -> (w591:refnum<vi>)
      n500 = control-ref of="Fine Tune Zone"() -> (w611:refnum<vi>)
      n501 = control-ref of="PID Delay (sec)"() -> (w610:refnum<vi>)
      n502 = control-ref of="Max_pos_limit"() -> (w609:refnum<vi>)
      n503 = control-ref of="Min_pos_limit"() -> (w608:refnum<vi>)
      n504 = control-ref of="i_limit"() -> (w607:refnum<vi>)
      n505 = control-ref of="pct_scale"() -> (w598:refnum<vi>)
      n506 = control-ref of="Deadband"() -> (w606:refnum<vi>)
      n507 = control-ref of="Kd"() -> (w605:refnum<vi>)
      n508 = control-ref of="Ki"() -> (w604:refnum<vi>)
      n509 = control-ref of="Kp"() -> (w603:refnum<vi>)
      n510 = control-ref of="Current Position"() -> (w602:refnum<vi>)
      n511 = control-ref of="Set Load"() -> (w601:refnum<vi>)
      n512 = control-ref of="Current Load"() -> (w600:refnum<vi>)
      n513 = control-ref of="Pulse delta"() -> (w599:refnum<vi>)
      n514 = control-ref of="Init Step"() -> (w597:refnum<vi>)
      n515 = control-ref of="Max Step Linit"() -> (w596:refnum<vi>)
      n516 = control-ref of="min_deadband_floor"() -> (w595:refnum<vi>)
      n517 = control-ref of="dynamic_spindle_noise_scalar"() -> (w594:refnum<vi>)
      n518 = control-ref of="min_finetune_floor"() -> (w593:refnum<vi>)
      n519 = control-ref of="filter_alpha"() -> (w592:refnum<vi>)
